vi "FilterVIDependencies.vi"(8 "error in (no error)":errorcluster, 9 "Dependency Paths":path[](array[path]), 10 "Dependency Names in":string[](array[string]), 11 "VI Name":string) -> (0 "error out":errorcluster, 1 "VIName":string, 2 "Dependency output paths":string[](array[string]), 3 "Dependency names out":string[](array[string]))   [LabVIEW 2017]
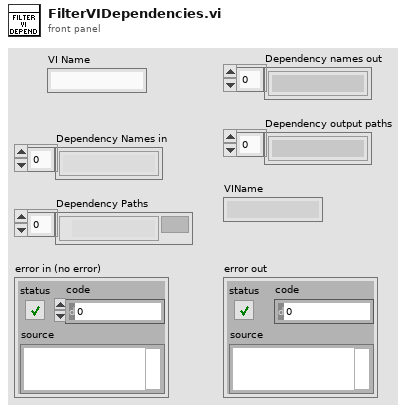
[diagram p1: front panel]
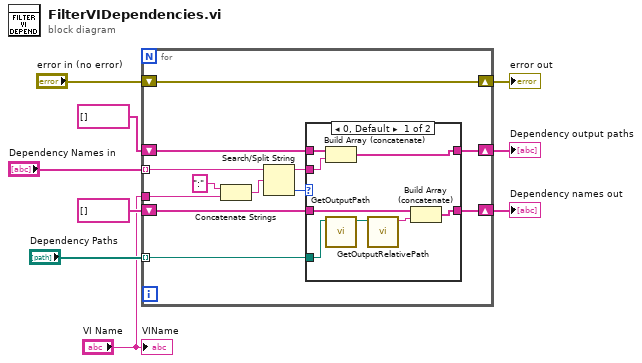
[diagram p0: block diagram]
diagram:
  n1 = for {
    tunnel: "VI Name" -> [w12]
    tunnel: "Dependency Names in" -> [w20] mode=indexing
    tunnel: "Dependency Paths" -> [w14] mode=indexing
    shift-right: [w18] -> w2
    shift-left: string[] [] ("Dependency Names") -> [w19]
    shift-right: [w16] -> w1
    shift-left: string[] [] ("Dependency Names") -> [w17]
    shift-right: [w15] -> w4
    shift-left: "error in (no error)" -> [w15]
    n2 = Concatenate Strings(":" ("string"), w12) -> (w11:string)
    n3 = Search/Split String(string=w20, search string/char (-)=w11) -> (substring before match=w13:string, offset of match=w21:i32)  [unwired: 1 in, 1 out]
    n4 = case shown="0, Default" w21 {
      tunnel: w13 -> [w29 _]
      tunnel: w19 -> [w28 w31]
      tunnel: [w27 w31] -> w18
      tunnel: w17 -> [w26 w30]
      tunnel: [w25 w30] -> w16
      tunnel: w14 -> [w23 _]
      frame 0, Default {
        n5 = Build Array (concatenate)(w28, w29) -> (w27:string[])
        n6 = call "GetOutputPath.vi"("Path"=w23) -> ("Output Path"=w24:path)  [unwired: 10 in]
        n7 = call "GetOutputRelativePath.vi"("Path"=w24) -> ("Output relative path"=w22:string)  [unwired: 9 in, 1 out]
        n8 = Build Array (concatenate)(w26, w22) -> (w25:string[])
      }
      frame -1 {
      }
    }
  }
  "Dependency names out" <- w1
  "Dependency output paths" <- w2
  "error out" <- w4
  "VIName" <- "VI Name"
